vi "ExSubCollectDisplayStore.vi"(3 "error in (no error)":errorcluster, 4 "Store flag":i8, 5 "Display Title":string, 6 "Handle Cluster":T1) -> (0 "error out":errorcluster, 1 "got frame":u32, 2 "Handle Cluster Out":T1)   [LabVIEW 2010]
panel:
  # "ExSubCollectDisplayStore:\nThis sub-VI checks to see if data has arrived from camera,\nif so it then puts it in image object and displays it. If store \nswitch is set it will also store it."
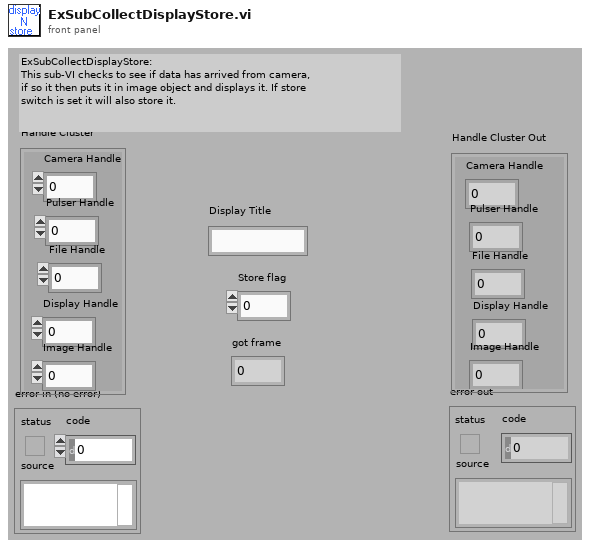
[diagram p1: front panel]
types:
  T1 = cluster{"Camera Handle":u32, "Pulser Handle":u32, "File Handle":u32, "Display Handle":u32, "Image Handle":u32}
  T2 = cluster{"Camera Handle":u32, "Pulser Handle":u32, "File Handle":u32, "Display Handle":u32, "Data Handle":u32}
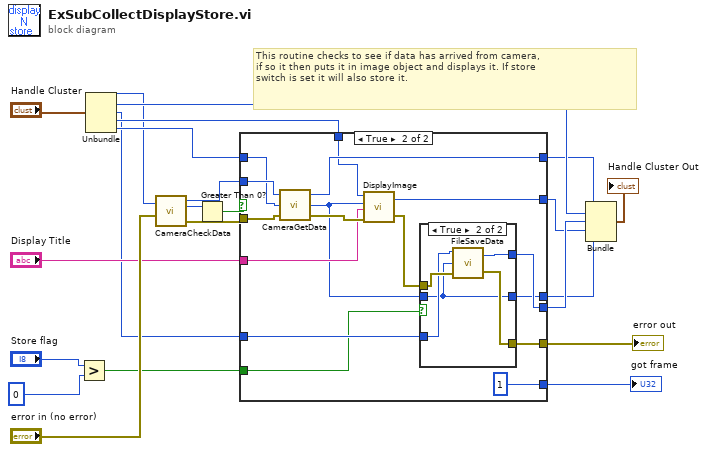
[diagram p0: block diagram]
diagram:
  # "This routine checks to see if data has arrived from camera,\nif so it then puts it in image object and displays it. If store \nswitch is set it will also store it."
  n1 = Greater?(x="Store flag", y=0) -> (0:w2:bool)
  n2 = Unbundle("Handle Cluster") -> ("Camera Handle"=w8:u32, "Pulser Handle"=w11:u32, "File Handle"=w12:u32, "Display Handle"=w14:u32, "Image Handle"=w15:u32)
  n3 = call <userlib>:"CameraCheckData.vi"("Camera Handle"=w8, "error in"="error in (no error)") -> ("Camera Handle"=w19:u32, "Number Of Frames Available"=w18:i32, "error out"=w17:errorcluster)
  n4 = Greater Than 0?(x=w18) -> (x > 0?=w20:bool)
  n5 = case shown="True" w20 {
    tunnel: w19 -> [w28 w44]
    tunnel: w17 -> [w27 w43]
    tunnel: w15 -> [w24 w38]
    tunnel: w14 -> [w26 w37]
    tunnel: [w28 w42] -> w9
    tunnel: [w25 w41] -> w7
    tunnel: "Display Title" -> [_ w36]
    tunnel: w12 -> [w25 w35]
    tunnel: [w26 w34] -> w6
    tunnel: [w27 w33] -> w10
    tunnel: [w24 w31] -> w5
    tunnel: w2 -> [_ w30]
    tunnel: [0 1] -> w1
    frame False {
    }
    frame True {
      n6 = call <userlib>:"CameraGetData.vi"("error in"=w43, "Data Handle"=w38, "Camera Handle"=w44) -> ("error out"=w40:errorcluster, "Data Handle"=w32:u32, "Camera Handle"=w42:u32)
      n7 = call <userlib>:"DisplayImage.vi"("error in"=w40, "Title"=w36, "Image Handle"=w32, "Display Handle"=w37) -> ("error out"=w39:errorcluster, "Display Handle"=w34:u32)
      n8 = case shown="True" w30 {
        tunnel: [w47 w52] -> w41
        tunnel: w39 -> [w46 w51]
        tunnel: w35 -> [w47 w49]
        tunnel: [w46 w50] -> w33
        tunnel: w32 -> [w45 w48]
        tunnel: [w45 w48] -> w31
        frame False {
        }
        frame True {
          n9 = call <userlib>:"FileSaveData.vi"("error in"=w51, "Image Handle"=w48, "File Handle"=w49) -> ("error out"=w50:errorcluster, "File Handle"=w52:u32)
        }
      }
    }
  }
  "error out" <- w10
  "got frame" <- w1
  n10 = Bundle("Camera Handle"=w9, "Pulser Handle"=w11, "File Handle"=w7, "Display Handle"=w6, "Data Handle"=w5) -> (→"Handle Cluster Out":T2)  [unwired: 1 in]
